vi "Configure Multi Eval Meas Power Scalar Enabled.vi"(8 "error in (no error)":errorcluster, 9 "Power Scalar (On)":bool=TRUE, 10 "Instance (1)":i32=1, 11 "VISA resource name":refnum<visa-resource-name>) -> (0 "error out":errorcluster, 3 "VISA resource name out":refnum<visa-resource-name>)   [LabVIEW 2015, in "Rohde&Schwarz CMP LR WPAN Measurement.lvlib"]
doc: "Enables or disables the evaluation of Power Scalar results in the multi-evaluation measurement.\n\nAttribute:\nRSCMPLRWM_ATTR_MULTIEVAL_POWER_SCALAR_ENABLED\n\nRemote-control command:\nCONFigure:WPAN:MEAS<i>:MEValuation:RESult:PSCalar"
uses:
  <instrlib>/Rohde&Schwarz CMP LR WPAN Measurement/Rohde&Schwarz CMP LR WPAN Measurement.lvlib
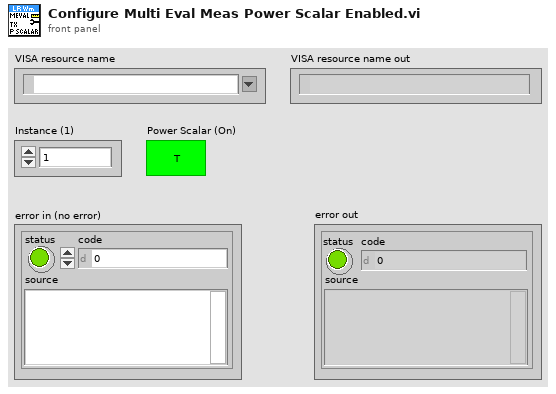
[diagram p1: front panel]
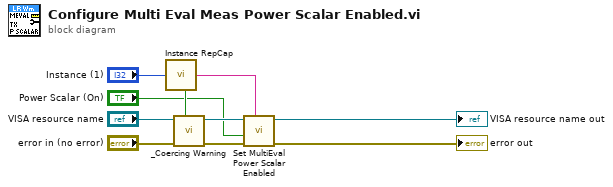
[diagram p0: block diagram]
diagram:
  n1 = call <instrlib>:"Instance RepCap.vi"("Instance In"="Instance (1)") -> ("In Range?"=w7:bool, "RepCap Identifier Out"=w8:string)  [unwired: 1 in]
  n2 = call <instrlib>:"_Coercing Warning.vi"("In Range?"=w7, "error in (no error)"="error in (no error)", "VISA resource name"="VISA resource name") -> ("error out"=w4:errorcluster, "VISA resource name out"=w3:refnum<visa-resource-name>)  [unwired: 7 in]
  n3 = call "Set MultiEval Power Scalar Enabled"("Repeated Capabilities"=w8, "error in (no error)"=w4, "MultiEval Power Scalar Enabled (OFF)"="Power Scalar (On)", "instrument handle"=w3) -> ("error out"=→"error out":errorcluster, "instrument handle out"=→"VISA resource name out":refnum<visa-resource-name>)  [unwired: 6 in]
